vi "Destroy.vi"(0 "reference in":refnum<class "debugging.lvclass">, 5 "error in (no error)":errorcluster) -> (14 "reference out":refnum<class "debugging.lvclass">, 19 "error out":errorcluster)   [LabVIEW 2019, in "debugging.lvclass"]
uses:
  debugging.lvclass
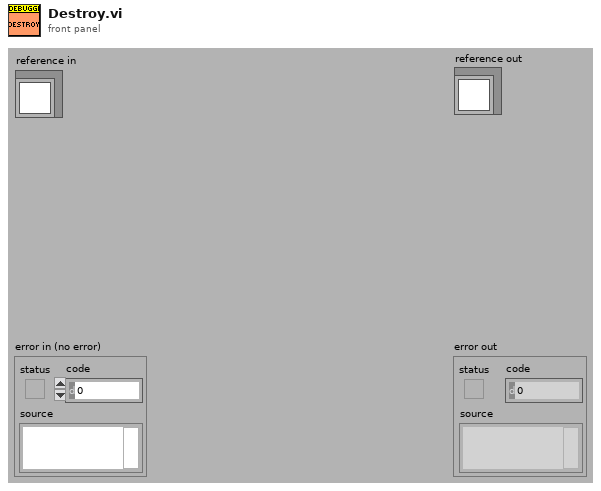
[diagram p1: front panel]
types:
  T1 = typedef "debugging.lvclass/ObjectAttributes.ctl" = cluster{"Attribute1":dbl}
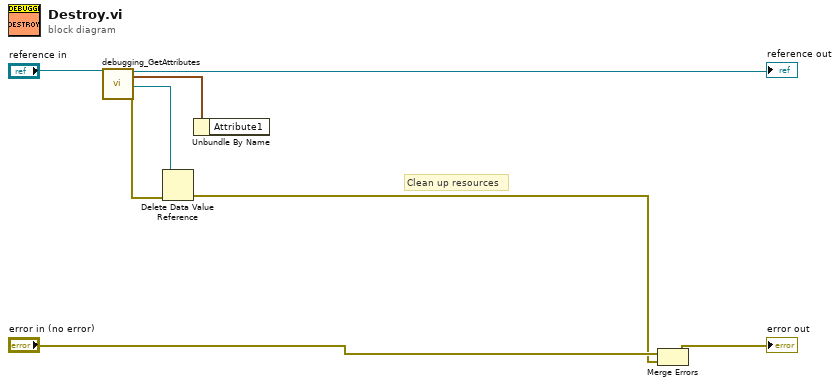
[diagram p0: block diagram]
diagram:
  # "Clean up resources"
  n1 = call "debugging_GetAttributes.vi"("reference in"="reference in") -> ("reference out"=→"reference out":refnum<class "debugging.lvclass">, "Data"=w3:T1, "DataRef"=w4:refnum<data-value>, "error out"=w5:errorcluster)  [unwired: 15 in]
  n2 = Delete Data Value Reference(data value reference=w4, error in=w5) -> (error out=w1:errorcluster)  [unwired: 1 out]
  n3 = Unbundle By Name(w3) -> ()  [unwired: 1 out]
  n4 = Merge Errors("error in (no error)", w1) -> (→"error out":errorcluster)
